vi "Clone Template.vi"() -> ()   [LabVIEW 2020]
panel:
  out "error out":errorcluster
  in  "base path":path
  in  "New Demo Name":string
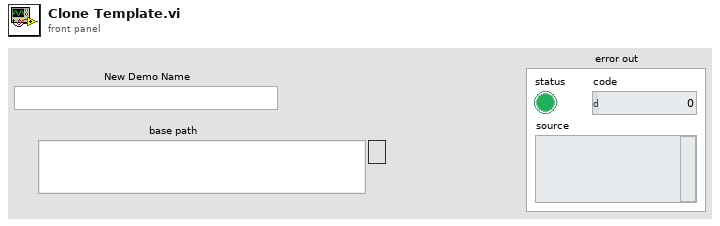
[diagram p1: front panel]
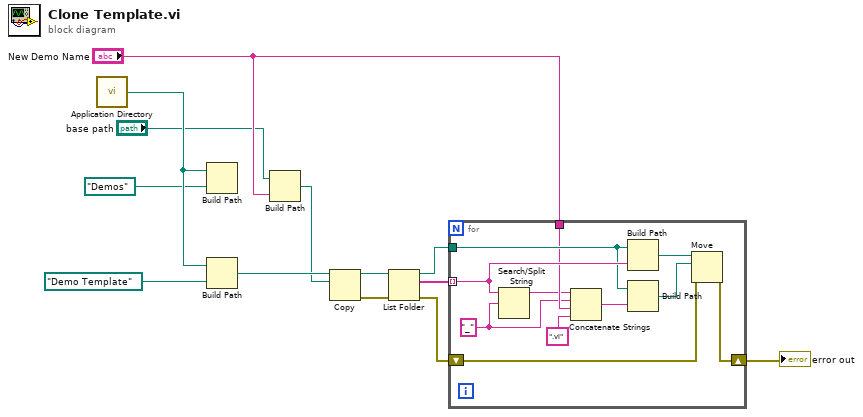
[diagram p0: block diagram]
diagram:
  n1 = call <vilib>:"Application Directory.vi"() -> ("Application Directory"=w12:path)
  n2 = Build Path(base path=w12, name or relative path=path "Demos" ("Path")) -> ()  [unwired: 1 out]
  n3 = Build Path(base path=w12, name or relative path=path "Demo Template" ("Path")) -> (appended path=w10:path)
  n4 = Build Path(base path="base path", name or relative path="New Demo Name") -> (appended path=w9:path)
  n5 = Copy(10:w9, 11:w10) -> (0:w1:errorcluster, 3:w8:path)  [unwired: 3 in, 1 out]
  n6 = List Folder(path=w8, error in=w1) -> (path out=w6:path, filenames=w7:string[], error out=w3:errorcluster)  [unwired: 2 in, 1 out]
  n7 = for {
    tunnel: w7 -> [w24] mode=indexing
    tunnel: w6 -> [w22]
    tunnel: "New Demo Name" -> [w21]
    shift-right: [w14] -> w2
    shift-left: w3 -> [w15]
    w17 = "_" ("search string/char (-)")
    n8 = Search/Split String(string=w24, search string/char (-)=w17) -> (substring before match=w16:string)  [unwired: 1 in, 2 out]
    n9 = Concatenate Strings(w16, w17, w21, ".vi" ("string")) -> (w19:string)
    n10 = Build Path(base path=w22, name or relative path=w24) -> (appended path=w23:path)
    n11 = Build Path(base path=w22, name or relative path=w19) -> (appended path=w20:path)
    n12 = Move(source path=w23, error in=w15, 10:w20) -> (error out=w14:errorcluster)  [unwired: 2 in, 2 out]
  }
  "error out" <- w2
